vi "(Un)tag Lines.vi"(4 "Set if match (T)\\Set it no match (F) [T]":bool=TRUE, 5 "Context [name]":T1=enum."name", 6 "Tag (T)\\Untag (F) [T]":bool=TRUE, 7 "String\\Regex [\"\"]":string, 8 "error in (no error)":errorcluster, 10 "Use Regex? [T]":bool=TRUE, 11 "Carya Config in":refnum<class "Carya Config.lvclass">) -> (0 "error out":errorcluster, 1 "context":string[](array[string]), 2 "Section names":string[](array[string]), 3 "Carya Config out":refnum<class "Carya Config.lvclass">)   [LabVIEW 2013, in "Carya Config.lvclass"]
doc: "Copyright 2018, Carya Automatisering, Wiebe Walstra."
uses:
  Carya Config.lvclass
  CConfig Object/Data.ctl
  CConfig Object/CConfig Object.lvclass
  CConfig Object/Set Query/Set Query.lvclass
  CConfig Object/Composite Query/Composite Query.lvclass
  CConfig Object/Add Results Query/Add Results Query.lvclass
  CConfig Object/Step In Query/Step In Query.lvclass
  CConfig Object/Loop Query/Match Query/Match Query.lvclass
  CConfig Object/Loop Query/All Query/All Query.lvclass
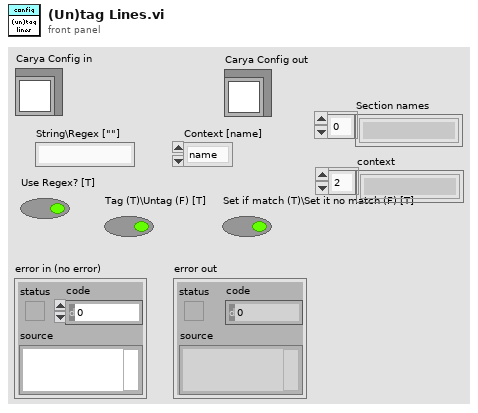
[diagram p1: front panel]
types:
  T1 = typedef "CConfig Object.lvclass/Data.ctl" = enum16{"pre", "name", "middle", "value", "post", "newline", "persistant", "tagged", "type"}
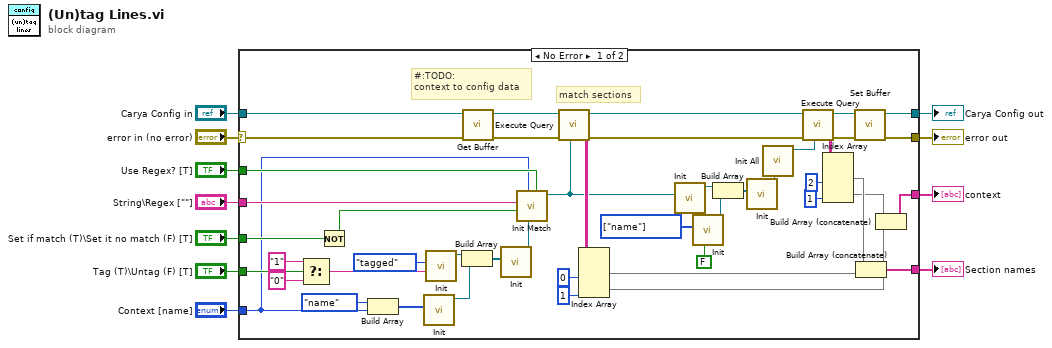
[diagram p0: block diagram]
diagram:
  n1 = case shown="No Error" "error in (no error)" {
    selector: "error in (no error)" -> [w50 w59]
    tunnel: [w52 w59] -> w10
    tunnel: [w53 w58] -> w8
    tunnel: "Carya Config in" -> [w56 w58]
    tunnel: "String\\Regex [\"\"]" -> [w57 _]
    tunnel: "Use Regex? [T]" -> [w24 _]
    tunnel: "Tag (T)\\Untag (F) [T]" -> [w55 _]
    tunnel: "Set if match (T)\\Set it no match (F) [T]" -> [w54 _]
    tunnel: "Context [name]" -> [w13 _]
    tunnel: [w16 _] -> w2
    tunnel: [w21 _] -> w1
    frame No Error {
      w28 = T1[] [enum."name"] items=["pre", "name", "middle", "value", "post", "newline", "persistant", "tagged", "type"] ("Data")
      # "match sections"
      # "#:TODO:\ncontext to config data"
      n2 = Select(t="1" ("Value"), s=w55, f="0") -> (s? t:f=w30:string)
      n3 = Not(x=w54) -> (.not. x?=w23:bool)
      n4 = Build Array(Data."name" ("Data [name]"), w13) -> (w20:T1[])
      n5 = call "Init.vi"("Data [name]"=w20) -> ("Find First Query out"=w43:refnum<class "Add Results Query.lvclass">)  [unwired: 9 in, 1 out]
      n6 = call "Init.vi"("Value"=w30, "Data [value]"=Data."tagged" ("Data")) -> ("Set Query out"=w45:refnum<class "Set Query.lvclass">)  [unwired: 8 in, 1 out]
      n7 = Build Array(w45, w43) -> (w44:refnum<class "CConfig Query.lvclass">[])
      n8 = call-dynamic "Get Buffer.vi"("error in (no error)"=w50, "Carya Config in"=w56) -> ("error out"=w49:errorcluster, "Config"=w48:refnum<class "Carya Config.lvclass">)  [unwired: 8 in]
      n9 = call "Init.vi"("Queries"=w44) -> ("Step In Query out"=w29:refnum<class "CConfig Query.lvclass">)  [unwired: 9 in, 1 out]
      n10 = call "Init Match.vi"("Regex [F]"=w24, "Found"=w29, "Data [name]"=w13, "Invert [F]"=w23, "Data"=w57) -> ("Find First Query out"=w14:refnum<class "Loop Query.lvclass">)  [unwired: 5 in, 1 out]
      n11 = call-dynamic "Execute Query.vi"("Config Query in"=w14, "error in (no error)"=w49, "Carya Config in"=w48) -> ("error out"=w34:errorcluster, "Results"=w26:string[][], "Carya Config out"=w33:refnum<class "Carya Config.lvclass">)  [unwired: 4 in, 2 out]
      n12 = Index Array(array=w26, index (col) #1=0 ("index (col)"), index (col) #2=1 ("index (col)")) -> (element #1=w25:string[], element #2=w15:string[])  [unwired: 2 in]
      n13 = call "Init.vi"("Config Query"=w14) -> ("Step In Query out"=w36:refnum<class "Step In Query.lvclass">)  [unwired: 9 in, 1 out]
      n14 = call "Init.vi"("Concatenate\\Build [T, Concatenate]"=FALSE ("Concatenate\\Build [T, Concatenate]"), "Data [name]"=w28) -> ("Find First Query out"=w40:refnum<class "Add Results Query.lvclass">)  [unwired: 8 in, 1 out]
      n15 = Build Array(w36, w40) -> (w35:refnum<class "CConfig Query.lvclass">[])
      n16 = call "Init.vi"("Queries"=w35) -> ("Step In Query out"=w37:refnum<class "CConfig Query.lvclass">)  [unwired: 9 in, 1 out]
      n17 = call "Init All.vi"("Found"=w37) -> ("Find First Query out"=w12:refnum<class "All Query.lvclass">)  [unwired: 9 in, 1 out]
      n18 = call-dynamic "Execute Query.vi"("Config Query in"=w12, "error in (no error)"=w34, "Carya Config in"=w33) -> ("error out"=w51:errorcluster, "Results"=w41:string[][], "Carya Config out"=w47:refnum<class "Carya Config.lvclass">)  [unwired: 4 in, 2 out]
      n19 = Index Array(array=w41, index (col) #1=2 ("disabled index (col)"), index (col) #2=1 ("index (col)")) -> (element #1=w22:string[], element #2=w17:string[])  [unwired: 2 in]
      n20 = call-dynamic "Set Buffer.vi"("error in (no error)"=w51, "Carya Config"=w47) -> ("error out"=w52:errorcluster, "Carya Config out"=w53:refnum<class "Carya Config.lvclass">)  [unwired: 8 in]
      n21 = Build Array (concatenate)(w22, w25) -> (w21:string[])
      n22 = Build Array (concatenate)(w17, w15) -> (w16:string[])
    }
    frame Error {
    }
  }
  "error out" <- w10
  "Carya Config out" <- w8
  "Section names" <- w1
  "context" <- w2
